vi "Enqueue ActorRef.vi"(8 "error in (no error)":errorcluster, 9 "UIRef":refnum<class "Message Enqueuer.lvclass">, 11 "Core in":refnum<class "Core.lvclass">) -> (0 "error out":errorcluster, 3 "Core out":refnum<class "Core.lvclass">)   [LabVIEW 2019, in "Core.lvlib" / "Core.lvclass"]
uses:
  Core.lvclass
  C:/Program Files (x86)/National Instruments/LabVIEW 2019/vi.lib/ActorFramework/Actor/Actor.lvclass
  C:/Projekty/_Wewnetrzne/PC_ActorFramework/07_Program/LABVIEW/02_Source/Modules/ModuleAbstract/ModuleAbstract.lvclass
  <vilib>/ActorFramework/Message Enqueuer/Message Enqueuer.lvclass
  <vilib>/ActorFramework/Actor/Actor.lvclass/Actor.ctl
  <vilib>/ActorFramework/Message Enqueuer/Message Enqueuer.lvclass/Message Enqueuer.ctl
  ModuleAbstract/ModuleAbstract.lvclass/ModuleAbstract.ctl
  Containers/ActorRefContainer/ActorRefContainer.lvclass/ActorRefContainer.ctl
  <vilib>/ActorFramework/Message Enqueuer/Init from Existing Queue.vi
  Containers/ActorRefContainer/ActorRefContainer.lvclass
  ModuleAbstract/ModuleAbstract.lvclass
  <vilib>/ActorFramework/Actor/Actor.lvclass
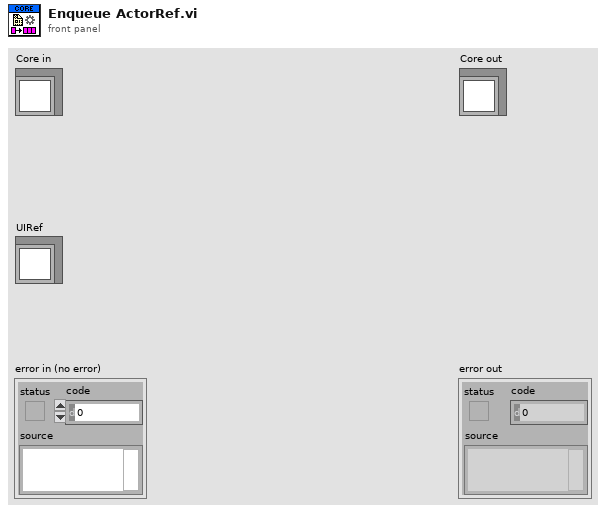
[diagram p1: front panel]
types:
  T1 = cluster{"ModRef":refnum<class "Message Enqueuer.lvclass">, "UIRef":refnum<class "Message Enqueuer.lvclass">}
  T2 = cluster{"Self Enqueuer":refnum<class "Message Enqueuer.lvclass">, "UIRef":refnum<class "Message Enqueuer.lvclass">}
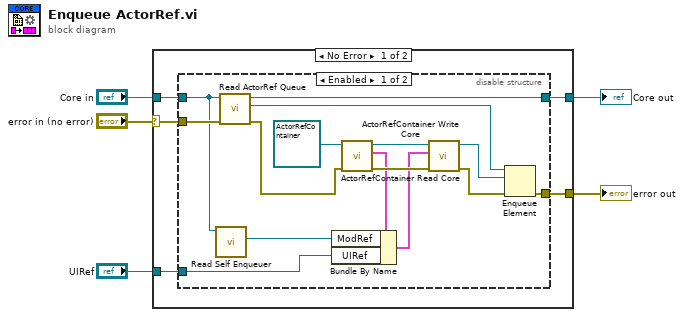
[diagram p0: block diagram]
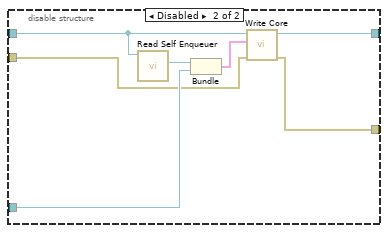
[diagram p2: hidden frame]
diagram:
  n1 = case shown="No Error" "error in (no error)" {
    selector: "error in (no error)" -> [w9 w34]
    tunnel: [w8 w34] -> w5
    tunnel: [w10 w33] -> w4
    tunnel: "Core in" -> [w6 w33]
    tunnel: "UIRef" -> [w7 _]
    frame No Error {
      n2 = disable-structure shown="Enabled" {
        disable-tunnel: [w25 w32] -> w10
        disable-tunnel: w9 -> [w24 w27]
        disable-tunnel: [w22 w26] -> w8
        disable-tunnel: w7 -> [w13 w30]
        disable-tunnel: w6 -> [w11 w28]
        frame Enabled {
          n3 = call <vilib>:"Read Self Enqueuer.vi"("Actor"=w11) -> ("Self Enqueuer"=w12:refnum<class "Message Enqueuer.lvclass">)  [unwired: 10 in]
          n4 = call "Read ActorRef Queue.vi"("error in (no error)"=w24, "ModuleAbstract in"=w11) -> ("error out"=w19:errorcluster, "ActorRef Queue"=w23:refnum<queue>, "ModuleAbstract out"=w25:refnum<class "Core.lvclass">)  [unwired: 7 in]
          n5 = call "ActorRefContainer Read Core.vi"("error in (no error)"=w19, "ActorRefContainer in"=refnum<class "ActorRefContainer.lvclass"> refnum ("ActorRefContainer")) -> ("error out"=w18:errorcluster, "Core"=w15:T1, "ActorRefContainer out"=w20:refnum<class "ActorRefContainer.lvclass">)  [unwired: 7 in]
          n6 = Bundle By Name(cluster=w15, "ModRef"=w12, "UIRef"=w13) -> (w14:T1)
          n7 = call "ActorRefContainer Write Core.vi"("error in (no error)"=w18, "Core"=w14, "ActorRefContainer in"=w20) -> ("error out"=w17:errorcluster, "ActorRefContainer out"=w16:refnum<class "ActorRefContainer.lvclass">)  [unwired: 7 in]
          n8 = Enqueue Element(queue=w23, element=w16, error in (no error)=w17) -> (error out=w22:errorcluster)  [unwired: 1 in, 2 out]
        }
        frame Disabled {
          n9 = call <vilib>:"Read Self Enqueuer.vi"("Actor"=w28) -> ("Self Enqueuer"=w31:refnum<class "Message Enqueuer.lvclass">)  [unwired: 10 in]
          n10 = Bundle("Self Enqueuer"=w31, "UIRef"=w30) -> (w29:T2)  [unwired: 1 in]
          n11 = call "Write Core.vi"("error in (no error)"=w27, "Core"=w29, "ModuleAbstract in"=w28) -> ("error out"=w26:errorcluster, "ModuleAbstract out"=w32:refnum<class "Core.lvclass">)  [unwired: 7 in]
        }
      }
    }
    frame Error {
    }
  }
  "error out" <- w5
  "Core out" <- w4
